vi "AdaptToInputs.vi"(3 "Term Types":T1, 4 "XRef":refnum<vi>, 5 "State In":T5) -> (0 "Reply":string[](array[string]), 2 "State Out":T5)   [LabVIEW 2012, in "OpenG Empty Array.xnode"]
uses:
  OpenG Empty Array.xnode
  State.ctl
  <vilib>/XNodeSupport/XNodeTermTypeIDPairs.ctl
  <vilib>/XNodeSupport/XNodeTermTypeIDPair.ctl
  <vilib>/XNodeSupport/XNodeType.ctl
  <vilib>/XNodeSupport/XNodeString.ctl
  <userlib>/_LAVAcr/Scripting Tools/XNode Support/Find term type by ID_type.vi
  <userlib>/_LAVAcr/Scripting Tools/XNode Support/XNode Support.lvlib
  <vilib>/XNodeSupport/NI_XNodeSupport.lvlib
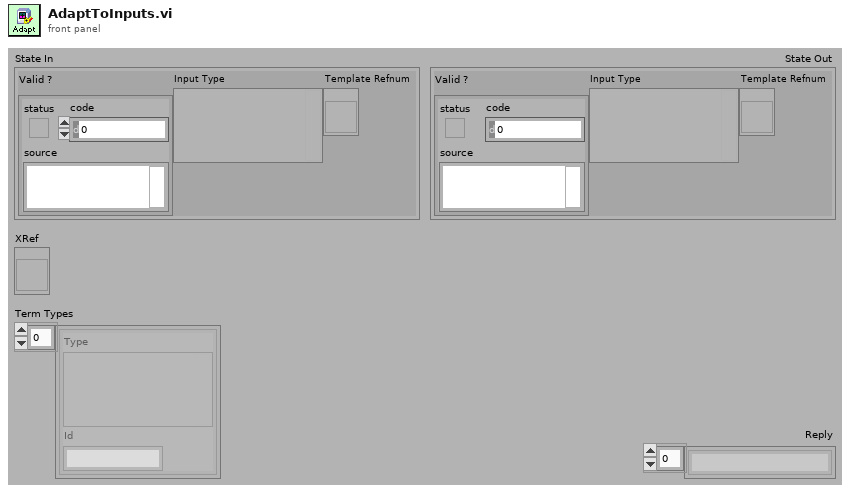
[diagram p1: front panel]
types:
  T1 = typedef "NI_XNodeSupport.lvlib/XNodeTermTypeIDPairs.ctl" = T2[]
  T2 = typedef "NI_XNodeSupport.lvlib/XNodeTermTypeIDPair.ctl" = cluster{"Type":T3, "Id":T4}
  T3 = typedef "NI_XNodeSupport.lvlib/XNodeType.ctl" = variant
  T4 = typedef "NI_XNodeSupport.lvlib/XNodeString.ctl" = string
  T5 = typedef "OpenG Empty Array.xnode/State.ctl" = cluster{"Valid ?":errorcluster, "Input Type":variant, "Template Refnum":refnum<vi>}
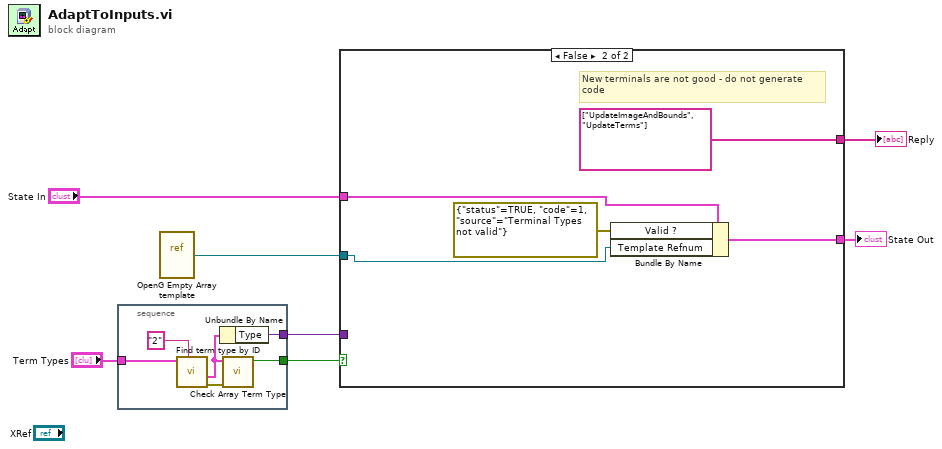
[diagram p0: block diagram]
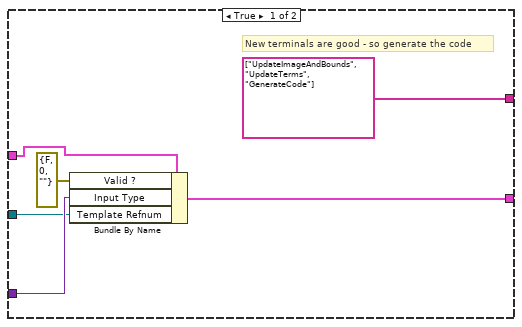
[diagram p2: hidden frame]
diagram:
  n1 = stacked-sequence {
    tunnel: "Term Types" -> [w13]
    tunnel: [w10] -> w6
    tunnel: [w8] -> w2
    frame #0 {
      n2 = call-poly <userlib>:"Find term type by ID.vi"("Search ID"="2", "Term Types"=w13) -> ("error out"=w11:errorcluster, "Term Type"=w9:T2)  [unwired: 1 in, 7 out]
      n3 = Unbundle By Name(w9) -> ("Type"=w8:T3)
      n4 = call <userlib>:"Check Array Term Type.vi"("error in (no error)"=w11, "Term Type"=w9) -> ("Is Good ?"=w10:bool)  [unwired: 3 in, 6 out]
    }
  }
  n5 = vi-ref "OpenG Empty Array template.vi"() -> (w1:refnum<vi>)
  n6 = case shown="False" w6 {
    tunnel: "State In" -> [w19 w24]
    tunnel: [w17 w22] -> w4
    tunnel: [string[] ["UpdateImageAndBounds", "UpdateTerms", "GenerateCode"] ("Reply") string[] ["UpdateImageAndBounds", "UpdateTerms"] ("Reply")] -> w3
    tunnel: w2 -> [w15 _]
    tunnel: w1 -> [w14 w20]
    frame True {
      # "New terminals are good - so generate the code"
      n7 = Bundle By Name(cluster=w19, "Valid ?"=errorcluster {"status"=FALSE, "code"=0, "source"=""}, "Input Type"=w15, "Template Refnum"=w14) -> (w17:T5)
    }
    frame False {
      # "New terminals are not good - do not generate\ncode"
      n8 = Bundle By Name(cluster=w24, "Valid ?"=errorcluster {"status"=TRUE, "code"=1, "source"="Terminal Types not valid"}, "Template Refnum"=w20) -> (w22:T5)
    }
  }
  "Reply" <- w3
  "State Out" <- w4
